vi "全局 数据数组大小.vi"() -> ()   [LabVIEW 2016, in "数据传输系统-06.lvlib"]
panel:
  out "分包标准":i32=3
  out "当前包号":i32
  out "总包数":i32
  out "数据数组大小":i32
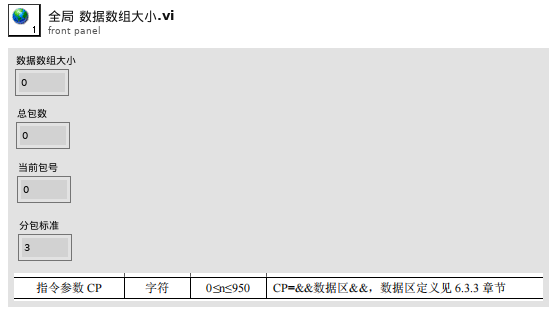
[diagram p1: front panel]
diagram:
